vi "DQMH_close modules.vi"(11 "Modules":T1) -> ()   [LabVIEW 2025]
uses:
  Libraries/USB IO/USB IO.lvlib
  Libraries/Power Supply/Power Supply.lvlib
  Libraries/Motor/Motor.lvlib
  Libraries/Wheatstone Bridge/Wheatstone Bridge.lvlib
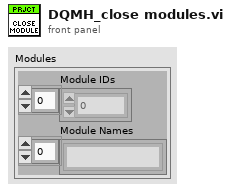
[diagram p1: front panel]
types:
  T1 = cluster{"Module IDs":i32[], "Module Names":string[]}
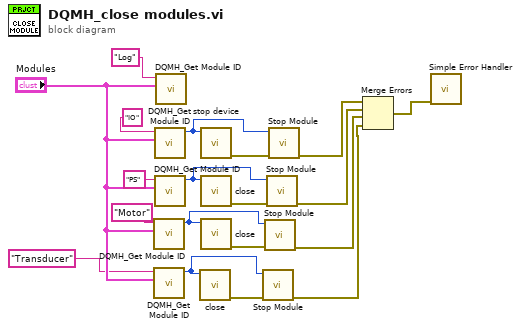
[diagram p0: block diagram]
diagram:
  n1 = call "DQMH_Get Module ID.vi"("Modules"="Modules", "Module Name"="Motor") -> ("Module ID out"=w6:i32)  [unwired: 9 in]
  n2 = call "DQMH_Get Module ID.vi"("Modules"="Modules", "Module Name"="Transducer") -> ("Module ID out"=w1:i32)  [unwired: 9 in]
  n3 = call "DQMH_Get Module ID.vi"("Modules"="Modules", "Module Name"="IO") -> ("Module ID out"=w14:i32)  [unwired: 9 in]
  n4 = call "DQMH_Get Module ID.vi"("Modules"="Modules", "Module Name"="PS") -> ("Module ID out"=w11:i32)  [unwired: 9 in]
  n5 = call "DQMH_Get Module ID.vi"("Modules"="Modules", "Module Name"="Log") -> ()  [unwired: 9 in, 1 out]
  n6 = call "close.vi"("Module ID"=w1) -> ("error out"=w2:errorcluster)  [unwired: 9 in, 1 out]
  n7 = call "stop device.vi"("Module ID"=w14) -> ("error out"=w15:errorcluster)  [unwired: 9 in, 1 out]
  n8 = call "close.vi"("Module ID"=w11) -> ("error out"=w12:errorcluster)  [unwired: 9 in, 1 out]
  n9 = call "close.vi"("Module ID"=w6) -> ("error out"=w5:errorcluster)  [unwired: 9 in, 1 out]
  n10 = call "Stop Module.vi"("error in"=w2, "Module ID"=w1) -> ("error out"=w3:errorcluster)  [unwired: 9 in]
  n11 = call "Stop Module.vi"("error in"=w5, "Module ID"=w6) -> ("error out"=w4:errorcluster)  [unwired: 9 in]
  n12 = call "Stop Module.vi"("error in"=w12, "Module ID"=w11) -> ("error out"=w10:errorcluster)  [unwired: 9 in]
  n13 = call "Stop Module.vi"("error in"=w15, "Module ID"=w14) -> ("error out"=w16:errorcluster)  [unwired: 9 in]
  n14 = Merge Errors(w16, w10, w4, w3) -> (w18:errorcluster)
  n15 = call <vilib>:"Simple Error Handler.vi"("error in (no error)"=w18) -> ()  [unwired: 4 in, 5 out]
